vi "Read Result Received.vi"(8 "error in (no error)":errorcluster, 11 "WAMP Client in":refnum<class "WAMP Client.lvclass">) -> (0 "error out":errorcluster, 2 "Result Received":refnum<user-event>, 3 "WAMP Client out":refnum<class "WAMP Client.lvclass">)   [LabVIEW 2020, in "wamplv.lvlib" / "WAMP Client.lvclass"]
uses:
  <userlib>/wamplv/WAMP Client/WAMP Client.lvclass
  <userlib>/wamplv/WAMP Client/TypeDef/RESULT Payload.ctl
  <userlib>/wamplv/WAMP Client/TypeDef/WAMP Error Payload.ctl
  <userlib>/wamplv/WAMP Client/WAMP Client.lvclass/WAMP Client.ctl
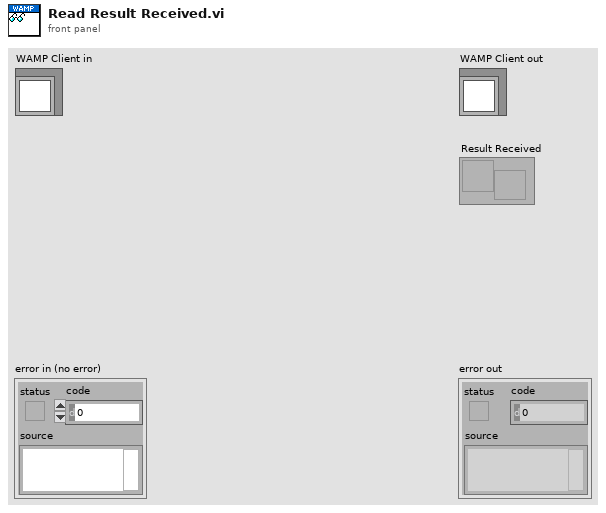
[diagram p1: front panel]
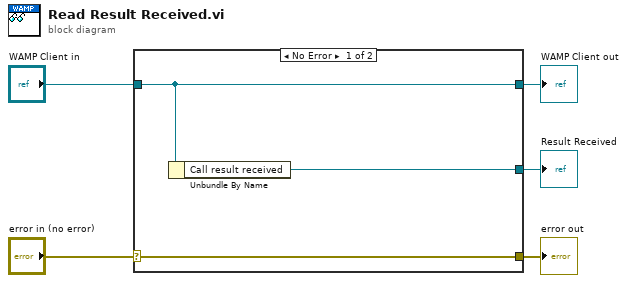
[diagram p0: block diagram]
diagram:
  n1 = case shown="No Error" "error in (no error)" {
    selector: "error in (no error)" -> [w8 w9]
    tunnel: [w8 w9] -> w4
    tunnel: [w7 w10] -> w2
    tunnel: "WAMP Client in" -> [w7 w10]
    tunnel: [w6 _] -> w1
    frame No Error {
      n2 = Unbundle By Name(w7) -> ("Call result received"=w6:refnum<user-event>)
    }
    frame Error {
    }
  }
  "error out" <- w4
  "WAMP Client out" <- w2
  "Result Received" <- w1
